vi "set_myMsgEvent.vi"(8 "error in (no error)":errorcluster, 10 "HGF_Event":refnum<class "HGF_Event.lvclass">, 11 "MoAgSy_AgentBase":refnum<class "MoAgSy_AgentBase.lvclass">) -> (0 "error out":errorcluster, 3 "MoAgSy_AgentBase":refnum<class "MoAgSy_AgentBase.lvclass">)   [LabVIEW 2009, in "MoAgSy_Base.lvlib" / "MoAgSy_AgentBase.lvclass"]
uses:
  MoAgSy_AgentBase.lvclass
  HGF_BaseClasses/HGF_Event/HGF_Event.lvclass
  MoAgSy_AgentBase.lvclass/MoAgSy_AgentBase.ctl
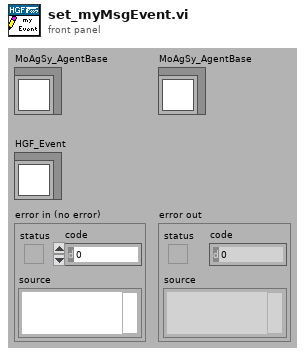
[diagram p1: front panel]
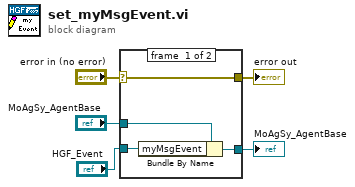
[diagram p0: block diagram]
diagram:
  n1 = case shown="No Error" "error in (no error)" {
    selector: "error in (no error)" -> [w9 w10]
    tunnel: [w9 w10] -> w4
    tunnel: [w7 w11] -> w2
    tunnel: "MoAgSy_AgentBase" -> [w8 w11]
    tunnel: "HGF_Event" -> [w6 _]
    frame #0 {
      n2 = Bundle By Name(cluster=w8, "myMsgEvent"=w6) -> (w7:refnum<class "MoAgSy_AgentBase.lvclass">)
    }
    frame #1 {
    }
  }
  "error out" <- w4
  "MoAgSy_AgentBase" <- w2
